vi "String_to String Array.vi"(8 "Allow Empty Tokens? (F)":bool, 9 "Put In Array If Found":string[](array[string]), 10 "Seperators (;)":string[](array[string]), 11 "Input String":string) -> (1 "Seperator Index Array Out":i32[](array[numeric]), 2 "String Array Out Blanks Removed Out":string[](array[string]), 3 "String Array Out":string[](array[string]))   [LabVIEW 2023]
uses:
  436d8972-33f1-43f4-ab8b-8338dfe66787.vi
  436d8972-33f1-43f4-ab8b-8338dfe66787.vi/4af5495f-31c7-4d59-8095-6cfc567fa6d4.vi
  436d8972-33f1-43f4-ab8b-8338dfe66787.vi/90930f07-b8e2-4d8c-a2d7-288f2fb4736d.vi
  436d8972-33f1-43f4-ab8b-8338dfe66787.vi/c0e9867c-5b49-4a19-9d71-73a29a90c073.vi
  436d8972-33f1-43f4-ab8b-8338dfe66787.vi/4af5495f-31c7-4d59-8095-6cfc567fa6d4.vi/42d3b4a4-cf10-4672-8650-5b246f1a6367.vi
  436d8972-33f1-43f4-ab8b-8338dfe66787.vi/90930f07-b8e2-4d8c-a2d7-288f2fb4736d.vi/b4c01bf9-b5f7-4610-85d9-f8261c7f5c83.vi
  436d8972-33f1-43f4-ab8b-8338dfe66787.vi/c0e9867c-5b49-4a19-9d71-73a29a90c073.vi/6868f419-8ba5-4c64-ad58-1d413efecb53.vi
  436d8972-33f1-43f4-ab8b-8338dfe66787.vi/c0e9867c-5b49-4a19-9d71-73a29a90c073.vi/7f435ff2-164e-468c-b25e-8feec744d60d.vi
  436d8972-33f1-43f4-ab8b-8338dfe66787.vi/c0e9867c-5b49-4a19-9d71-73a29a90c073.vi/25c58bee-37da-4e1e-86ad-284eaedd800c.vi
  436d8972-33f1-43f4-ab8b-8338dfe66787.vi/90930f07-b8e2-4d8c-a2d7-288f2fb4736d.vi/b4c01bf9-b5f7-4610-85d9-f8261c7f5c83.vi/3ce94938-5d63-4334-bea0-e8fce08a5599.vi
  String_Find many Strings.vi
panel:
  out "Seperated array":string[](array[string])
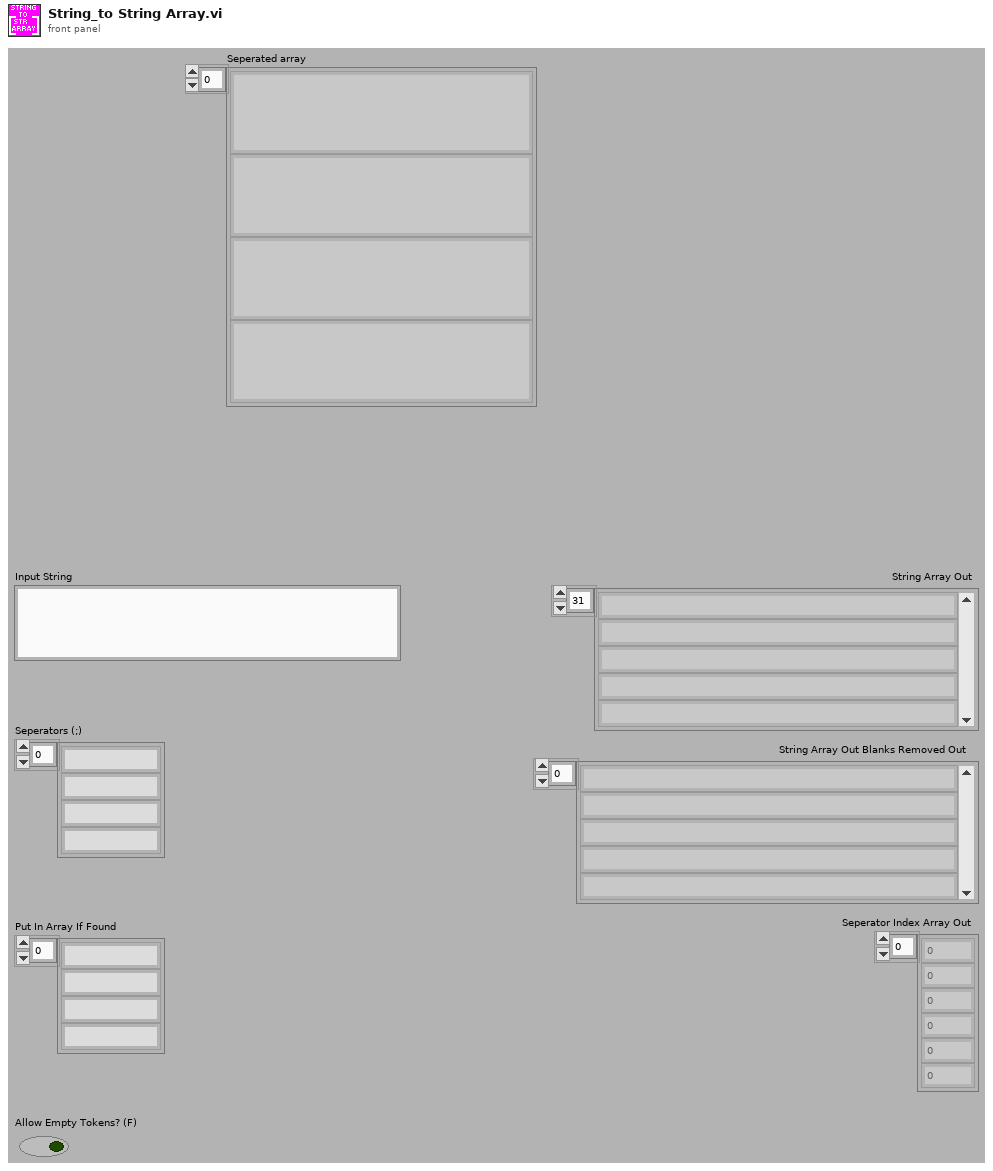
[diagram p1: front panel]
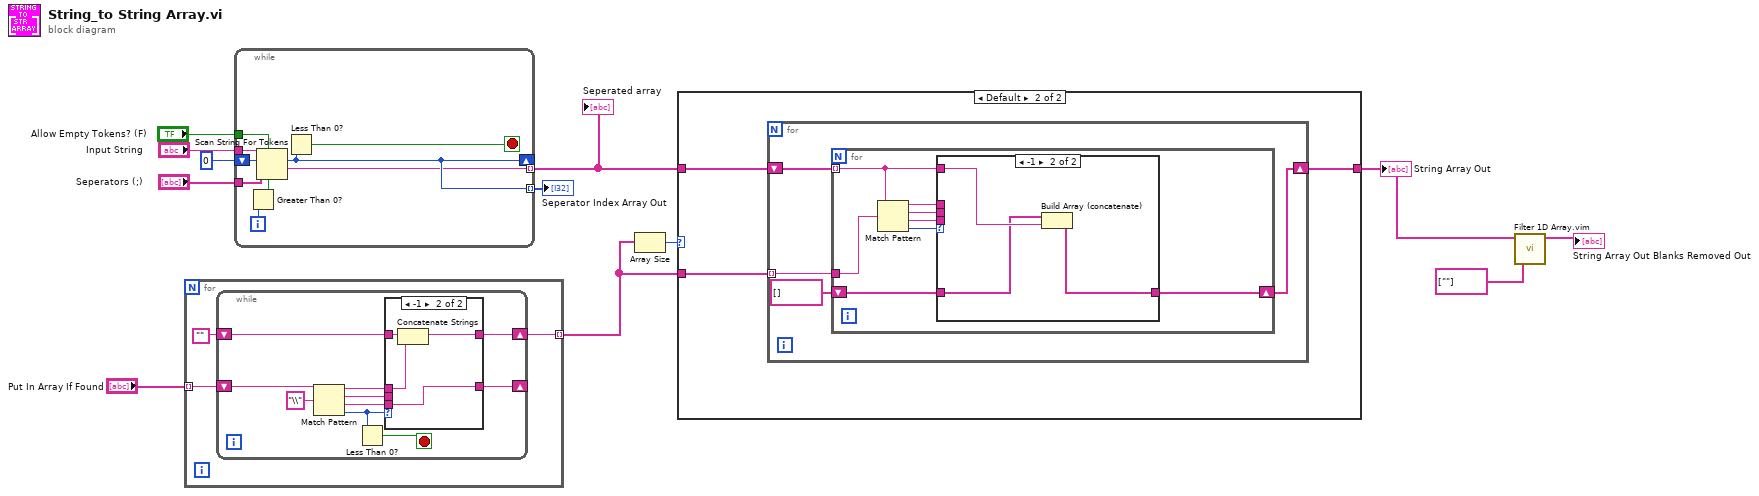
[diagram p0: block diagram]
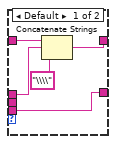
[diagram p2: hidden frame]
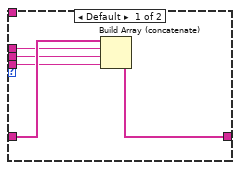
[diagram p4: hidden frame]
diagram:
  n1 = for {
    tunnel: "Put In Array If Found" -> [w15] mode=indexing
    tunnel: [w13] -> w4 mode=indexing
    n2 = while {
      shift-right: [w17] -> _
      shift-left: w15 -> [w25]
      shift-right: [w21] -> w13
      shift-left: "" -> [w22]
      stop <- w23 stop-if-true
      n3 = Match Pattern(string=w25, regular expression="\\") -> (before substring=w19:string, match substring=w18:string, after substring=w16:string, offset past match=w20:i32)  [unwired: 1 in]
      n4 = Less Than 0?(x=w20) -> (x < 0?=w23:bool)
      n5 = case shown="-1" w20 {
        tunnel: w22 -> [w28 w34]
        tunnel: [w29 w33] -> w21
        tunnel: w19 -> [w27 w32]
        tunnel: w18 -> [_ _]
        tunnel: [w30 w31] -> w17
        tunnel: w16 -> [w30 w31]
        frame Default {
          n6 = Concatenate Strings(w28, w27, "\\\\" ("regular expression")) -> (w29:string)
        }
        frame -1 {
          n7 = Concatenate Strings(w34, w32) -> (w33:string)
        }
      }
    }
  }
  n8 = while {
    tunnel: "Input String" -> [w43]
    tunnel: [w35] -> w7 mode=indexing
    shift-right: [w36] -> _
    shift-left: 0 ("offset past token") -> [w42]
    tunnel: "Seperators (;)" -> [w38]
    tunnel: "Allow Empty Tokens? (F)" -> [w37]
    tunnel: [w36] -> w8 mode=indexing
    i -> [w41]
    stop <- w39 stop-if-true
    n9 = Greater Than 0?(x=w41) -> (x > 0?=w40:bool)
    n10 = Scan String For Tokens(4:w40, 5:w37, 6:w38, 8:w42, 9:w43) -> (1:w35:string, 2:w36:i32)  [unwired: 1 in, 2 out]
    n11 = Less Than 0?(x=w36) -> (x < 0?=w39:bool)
  }
  "Seperator Index Array Out" <- w8
  "Seperated array" <- w7
  n12 = Array Size(array=w4) -> (size(s)=w6:i32)
  n13 = case shown="Default" w6 {
    tunnel: w7 -> [w44 w45]
    tunnel: w4 -> [_ w47]
    tunnel: [w44 w46] -> w3
    frame 0 {
    }
    frame Default {
      n14 = for {
        tunnel: w47 -> [w51] mode=indexing
        shift-right: [w50] -> w46
        shift-left: w45 -> [w49]
        n15 = for {
          tunnel: w49 -> [w58] mode=indexing
          tunnel: w51 -> [w59]
          shift-right: [w52] -> w50
          shift-left: string[] [] -> [w53]
          n16 = Match Pattern(string=w58, regular expression=w59) -> (before substring=w54:string, match substring=w55:string, after substring=w56:string, offset past match=w57:i32)  [unwired: 1 in]
          n17 = case shown="-1" w57 {
            tunnel: w58 -> [_ w67]
            tunnel: w56 -> [w62 _]
            tunnel: w55 -> [w61 _]
            tunnel: w54 -> [w60 _]
            tunnel: w53 -> [w64 w65]
            tunnel: [w63 w66] -> w52
            frame Default {
              n18 = Build Array (concatenate)(w64, w60, w61, w62) -> (w63:string[])
            }
            frame -1 {
              n19 = Build Array (concatenate)(w65, w67) -> (w66:string[])
            }
          }
        }
      }
    }
  }
  "String Array Out" <- w3
  n20 = call "Filter 1D Array.vim"("Items To Filter"=string[] [""] ("Items to Filter"), "Array"=w3) -> ("Filtered Array Out"=→"String Array Out Blanks Removed Out":string[])  [unwired: 4 in, 1 out]
